vi "Config Init.vi"(8 "error in (no error)":errorcluster, 11 "Path":path) -> (0 "error out":errorcluster)   [LabVIEW 2015]
uses:
  Configuration.ctl
  Support/Global Objects.vi
panel:
  in  "Configuration":T1={"Throttle Dead Zone"=0.05, "Throttle Ramp Rate"=0.05, "Turn Dead Zone"=0.05, "Auton"={"Motion Plan P"=0.2, "Motion Plan I"=0.02, "Motion Plan D"=0.05}, "Auto Upshift Enabled"=FALSE, "Upshift Min Throttle"=0.75, "Upshift Min Velocity"=8.0, "Min time before upshift"=200.0, "Shift Throttle Detent"=0, "Min time before downshift"=200.0, "Turn PID"={"Motion Plan P"=0.2, "Motion Plan I"=0.02, "Motion Plan D"=0.05}, "Auto Coast Downshift"=FALSE, "Downshift Coast Max Vel"=10.0, "Downshift Coast Throttle Epsilon"=0.1, "Left Motor Calibration"=1.0, "Right Motor Calibration"=1.0, "Tank Mode"=TRUE, "Shooter PID"={"Shooter  P"=0.01, "Shooter  I"=0.0, "Shooter  D"=0.0}}
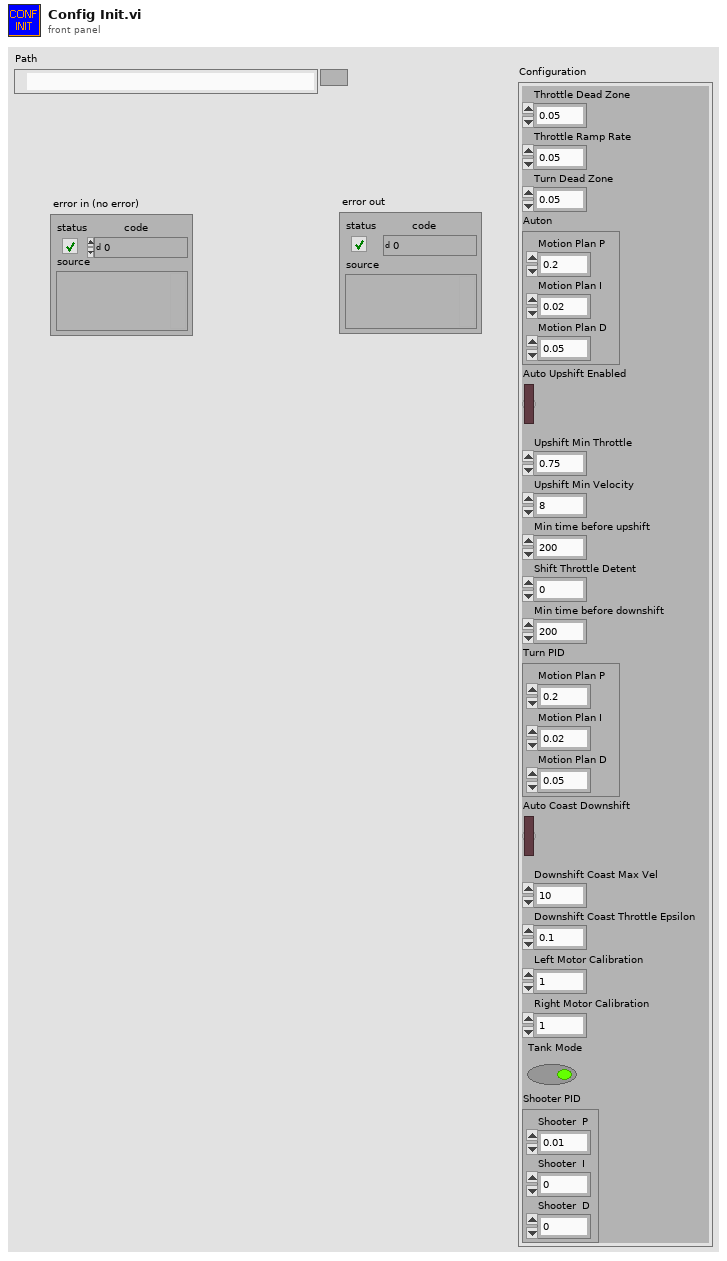
[diagram p1: front panel]
types:
  T1 = typedef "Configuration.ctl" = cluster{"Throttle Dead Zone":dbl, "Throttle Ramp Rate":dbl, "Turn Dead Zone":dbl, "Auton":cluster{"Motion Plan P":dbl, "Motion Plan I":dbl, "Motion Plan D":dbl}, "Auto Upshift Enabled":bool, "Upshift Min Throttle":dbl, "Upshift Min Velocity":dbl, "Min time before upshift":dbl, "Shift Throttle Detent":u32, "Min time before downshift":dbl, "Turn PID":cluster{"Motion Plan P":dbl, "Motion Plan I":dbl, "Motion Plan D":dbl}, "Auto Coast Downshift":bool, "Downshift Coast Max Vel":dbl, "Downshift Coast Throttle Epsilon":dbl, "Left Motor Calibration":dbl, "Right Motor Calibration":dbl, "Tank Mode":bool, "Shooter PID":cluster{"Shooter  P":dbl, "Shooter  I":dbl, "Shooter  D":dbl}}
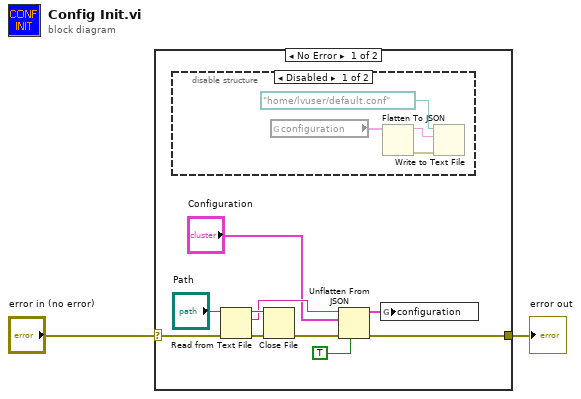
[diagram p0: block diagram]
diagram:
  n1 = case shown="No Error" "error in (no error)" {
    selector: "error in (no error)" -> [w11 w17]
    tunnel: [w4 w17] -> w1
    frame No Error {
      n2 = disable-structure shown="Disabled" {
        frame Disabled {
          n3 = global read "Global Objects.vi" "configuration"() -> (w16:T1)
          n4 = Flatten To JSON(anything=w16) -> (JSON string=w14:string, 11:w15:errorcluster)  [unwired: 2 in]
          n5 = Write to Text File(file (use dialog)=path "/home/lvuser/default.conf", text=w14, error in=w15) -> ()  [unwired: 1 in, 3 out]
        }
        frame Enabled {
        }
      }
      n6 = Read from Text File(file (use dialog)="Path", error in=w11) -> (refnum out=w10:refnum<file>, text=w8:string, error out=w9:errorcluster)  [unwired: 2 in, 1 out]
      n7 = Close File(refnum=w10, error in=w9) -> (error out=w5:errorcluster)  [unwired: 1 out]
      n8 = Unflatten From JSON(JSON string=w8, type and defaults="Configuration", default null elements? (F)=TRUE, error in (no error)=w5) -> (value=w3:T1, error out=w4:errorcluster)  [unwired: 3 in]
      n9 = global write "Global Objects.vi" "configuration"(w3) -> ()
    }
    frame Error {
    }
  }
  "error out" <- w1
